vi "GLOBAL CENTER FREQ.vi"(4 "Send OPC? (T)":bool=TRUE, 6 "READ ONLY (T)":bool, 7 "Delay  (ms)":i64=1 caption="Delay Time (s)", 8 "error in":errorcluster {"code" format="%.0x"}, 9 "Freq Units":u16(ring)=1 items=["Hz", "MHz", "GHz"], 10 "SET CF ()":dbl, 11 "Session In":refnum<visa-resource-name>="GPIB0::18::INSTR") -> (0 "error out":errorcluster {"code" format="%.0x"}, 2 "READ CF ()":string, 3 "Session Out":refnum<visa-resource-name>)   [LabVIEW 2018]
uses:
  Initialize References/Station References Global.vi
  Agilent MXA Series/Agilent MXA Series.lvlib
panel:
  out "RD(CMD)":string="FREQ:RF:CENT?"
  out "WR(CMD)":string
  out "IsPSA?(t)":bool
  in  "Timeout":u32=3000
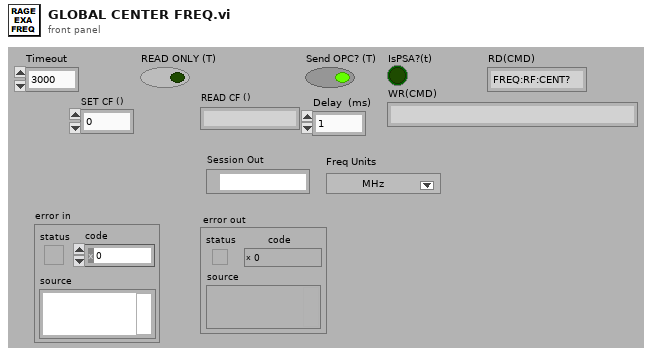
[diagram p1: front panel]
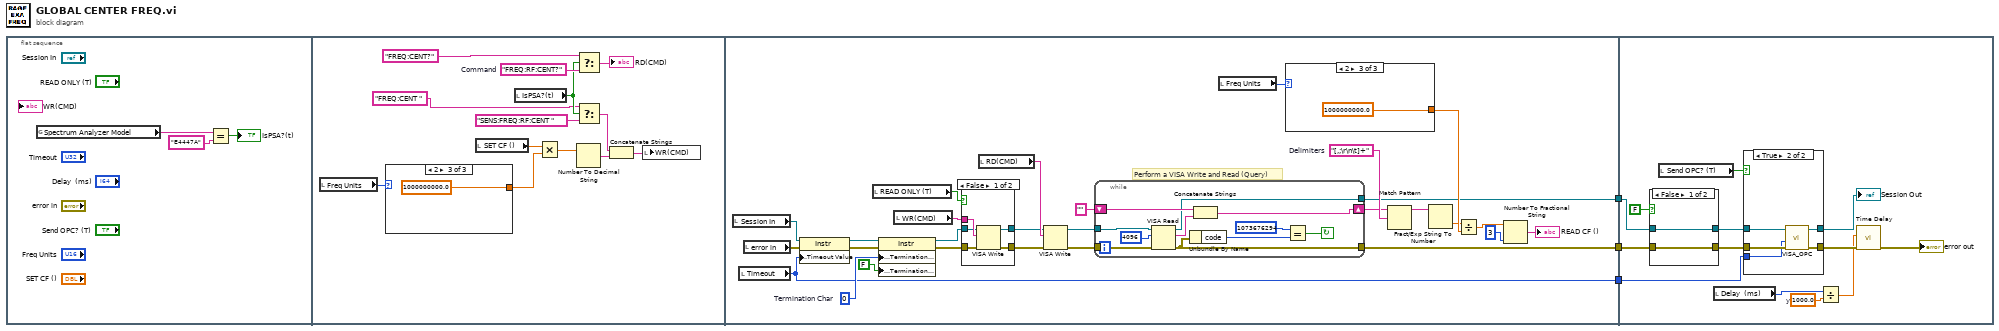
[diagram p0: block diagram]
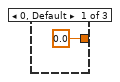
[diagram p2: hidden frame]
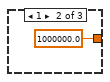
[diagram p3: hidden frame]
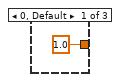
[diagram p4: hidden frame]
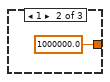
[diagram p5: hidden frame]
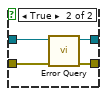
[diagram p8: hidden frame]
diagram:
  n1 = flat-sequence {
    tunnel: [w26] -> w3
    tunnel: [w25] -> w2
    tunnel: [w24] -> w1
    tunnel: w3 -> [w75]
    tunnel: w2 -> [w73]
    tunnel: w1 -> [w72]
    frame #0 {
      n2 = global read "Station References Global.vi" "Spectrum Analyzer Model"() -> (w6:string)
      n3 = Equal?(x=w6, y="E4447A") -> (x = y?=→"IsPSA?(t)":bool)
    }
    frame #1 {
      w10 = "FREQ:RF:CENT?"  # Command
      n4 = local read "Freq Units"() -> (w18:u16)
      n5 = case shown="2" w18 {
        tunnel: [0.0 ("y") 1000000.0 ("y") 1000000000.0 ("y")] -> w15
        frame 0, Default {
        }
        frame 1 {
        }
        frame 2 {
        }
      }
      n6 = local read "SET CF ()"() -> (w17:dbl)
      n7 = local read "IsPSA?(t)"() -> (w9:bool)
      n8 = Multiply(x=w17, y=w15) -> (x*y=w16:dbl)
      n9 = Select(t="FREQ:CENT?", s=w9, f=w10) -> (s? t:f=→"RD(CMD)":string)
      n10 = Select(t="FREQ:CENT ", s=w9, f="SENS:FREQ:RF:CENT " ("staticText")) -> (s? t:f=w12:string)
      n11 = Number To Decimal String(number=w16) -> (decimal integer string=w14:string)  [unwired: 1 in]
      n12 = Concatenate Strings(w12, w14) -> (w19:string)
      n13 = local write "WR(CMD)"(w19) -> ()
    }
    frame #2 {
      w30 = "[,;\r\n\t]+"  # Delimiters
      w28 = u8 0  # Termination Char
      # "Perform a VISA Write and Read (Query)"
      n14 = local read "Session In"() -> (w46:refnum<visa-resource-name>)
      n15 = local read "Timeout"() -> (w26:u32)
      n16 = local read "error in"() -> (w48:errorcluster)
      n17 = property class="Instr"(reference=w46, error in=w48, "General Settings:Timeout Value"=w26) -> (reference out=w34:refnum<visa-resource-name>, error out=w32:errorcluster)
      n18 = local read "READ ONLY (T)"() -> (w47:bool)
      n19 = property class="Instr"(reference=w34, error in=w32, "Message Based Settings:Termination Character"=w28, "Message Based Settings:Termination Character Enable"=FALSE ("enable")) -> (reference out=w38:refnum<visa-resource-name>, error out=w33:errorcluster)
      n20 = local read "WR(CMD)"() -> (w49:string)
      n21 = case shown="False" w47 {
        tunnel: w33 -> [w58 w59]
        tunnel: [w57 w59] -> w35
        tunnel: w49 -> [w56 _]
        tunnel: w38 -> [w55 w60]
        tunnel: [w54 w60] -> w39
        frame False {
          n22 = VISA Write(VISA resource name=w55, write buffer=w56, error in (no error)=w58) -> (VISA resource name out=w54:refnum<visa-resource-name>, error out=w57:errorcluster)  [unwired: 1 out]
        }
        frame True {
        }
      }
      n23 = local read "RD(CMD)"() -> (w50:string)
      n24 = VISA Write(VISA resource name=w39, write buffer=w50, error in (no error)=w35) -> (VISA resource name out=w36:refnum<visa-resource-name>, error out=w37:errorcluster)  [unwired: 1 out]
      n25 = while {
        tunnel: w36 -> [w68]
        shift-right: [w62] -> w23
        shift-left: "" -> [w67]
        tunnel: w37 -> [w65]
        tunnel: [w64] -> w24
        tunnel: [w61] -> w25
        stop <- w63 continue-if-true
        n26 = VISA Read(VISA resource name=w68, byte count=u32 4096 ("byte count (0)"), error in (no error)=w65) -> (VISA resource name out=w61:refnum<visa-resource-name>, read buffer=w66:string, error out=w64:errorcluster)  [unwired: 1 out]
        n27 = Unbundle By Name(w64) -> ("code"=w70:i32)
        n28 = Concatenate Strings(w67, w66) -> (w62:string)
        n29 = Equal?(x=1073676294, y=w70) -> (x = y?=w63:bool)
      }
      n30 = local read "Freq Units"() -> (w45:u16)
      n31 = case shown="2" w45 {
        tunnel: [1.0 ("y") 1000000.0 ("y") 1000000000.0 ("y")] -> w42
        frame 0, Default {
        }
        frame 1 {
        }
        frame 2 {
        }
      }
      n32 = Match Pattern(string=w23, regular expression=w30) -> (before substring=w40:string)  [unwired: 4 out]
      n33 = Fract/Exp String To Number(string=w40) -> (number=w41:dbl)  [unwired: 3 in, 1 out]
      n34 = Divide(x=w41, y=w42) -> (x/y=w43:dbl)
      n35 = Number To Fractional String(number=w43, precision (6)=i16 3) -> (F-format string=→"READ CF ()":string)  [unwired: 2 in]
    }
    frame #3 {
      w76 = 1000.0  # y
      n36 = case shown="False" FALSE {
        tunnel: w73 -> [w92 w97]
        tunnel: [w92 w96] -> w83
        tunnel: w72 -> [w93 w95]
        tunnel: [w93 w94] -> w84
        frame False {
        }
        frame True {
          n37 = call "Error Query.vi"("error in (no error)"=w95, "VISA resource name"=w97) -> ("error out"=w94:errorcluster, "VISA resource name out"=w96:refnum<visa-resource-name>)  [unwired: 6 in, 2 out]
        }
      }
      n38 = local read "Send OPC? (T)"() -> (w77:bool)
      n39 = local read "Delay  (ms)"() -> (w78:i64)
      n40 = case shown="True" w77 {
        tunnel: w84 -> [w85 w91]
        tunnel: w83 -> [w86 w90]
        tunnel: [w86 w89] -> w82
        tunnel: [w85 w88] -> w81
        tunnel: w75 -> [_ w87]
        frame False {
        }
        frame True {
          n41 = call "VISA_OPC.vi"("error in"=w91, "Timeout"=w87, "Session In"=w90) -> ("error out"=w88:errorcluster, "Session Out"=w89:refnum<visa-resource-name>)  [unwired: 6 in, 1 out]
        }
      }
      "Session Out" <- w82
      n42 = Divide(x=w78, y=w76) -> (x/y=w79:dbl)
      n43 = call "Time Delay"("error in (no error)"=w81, "Delay Time (s)"=w79) -> ("error out"=→"error out":errorcluster)  [unwired: 9 in]
    }
  }
